vi "Queue Is Nested.vi"(10 "Alias":string, 11 "Hello World Event in":refnum<class "Hello World Event.lvclass">) -> (2 "Queue Is Nested?":bool)   [LabVIEW 2021, in "Hello World Event.lvlib" / "Hello World Event.lvclass"]
uses:
  Hello World Event.lvclass
  Hello World Event.lvclass/Hello World Event.ctl
  jettl/Actor/Event Actor/Event Actor.lvclass
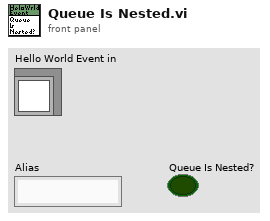
[diagram p1: front panel]
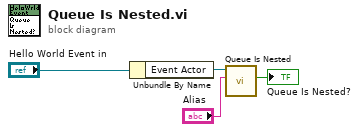
[diagram p0: block diagram]
diagram:
  n1 = Unbundle By Name("Hello World Event in") -> ("Event Actor"=w3:refnum<class "Event Actor.lvclass">)
  n2 = call-dynamic "Queue Is Nested.vi"("Alias"="Alias", "Actor in"=w3) -> ("Queue Is Nested?"=→"Queue Is Nested?":bool)  [unwired: 9 in]
